vi "Tuto_LED_réel.vi"   [LabVIEW 2018]
uses:
  <vilib>/rvi/Emulation/niFpgaGetClockAttributes.vi
  <vilib>/rvi/Emulation/niFpgaSctlEmulationGetInTimedLoop.vi
  <vilib>/rvi/Emulation/niFpgaEmulationReportErrorSimple.vi
  <vilib>/rvi/eio/common/nirviEmuTemplateMethod_errors.vi
  <vilib>/rvi/Emulation/niFpgaCriticalErrorInLSC.vi
  <vilib>/eio/EIONode/EIONode.xnode
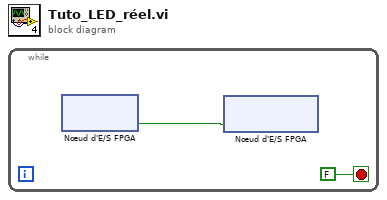
[diagram p0: block diagram]
diagram:
  n1 = while {
    stop <- FALSE stop-if-true
    n2 = xnode "Nœud d'E/S FPGA"() -> ("BTN0"=w2:bool)  [unwired: 1 in, 1 out]
    n3 = xnode "Nœud d'E/S FPGA"("BB3_DIO0"=w2) -> ()  [unwired: 1 in, 1 out]
  }
